vi "Test Write.vi"(8 "error in (no error)":errorcluster, 9 "data table":T1, 10 "data dictionary":refnum<class "data dictionary.lvclass">, 11 "runtime in":refnum<class "SystemLink File runtime.lvclass">) -> (0 "error out":errorcluster, 2 "Pass":bool[](array[boolean]), 3 "runtime out":refnum<class "SystemLink File runtime.lvclass">)   [LabVIEW 2015, in "SystemLink File Module tests.lvlib"]
uses:
  SystemLink File Module tests.lvlib
  module/execution/SystemLink File runtime.lvclass
  <vilib>/NI/Tag Bus/table/data table.ctl
  <vilib>/NI/Tag Bus/dictionary/data dictionary.lvclass
  module/execution/SystemLink File runtime.lvclass/SystemLink File runtime.ctl
  <vilib>/Skyline/Tag/Wrapper/Wrapper_class/NI Skyline Tag.lvclass/NI Skyline Tag.ctl
  <vilib>/NI/Tag Bus/dictionary/data dictionary.lvclass/data dictionary.ctl
  <vilib>/NI/Tag Bus/dictionary/lookup polymorphs/locate double.vi
  <vilib>/NI/Tag Bus/table/data polymorphs/write one/write Double.vi
  <vilib>/NI/Tag Bus/dictionary/lookup polymorphs/locate Single.vi
  <vilib>/NI/Tag Bus/table/data polymorphs/write one/write Single.vi
  <vilib>/NI/Tag Bus/dictionary/lookup polymorphs/locate I32.vi
  <vilib>/NI/Tag Bus/table/data polymorphs/write one/write I32.vi
  <vilib>/NI/Tag Bus/dictionary/lookup polymorphs/locate I16.vi
  <vilib>/NI/Tag Bus/table/data polymorphs/write one/write I16.vi
  <vilib>/NI/Tag Bus/dictionary/lookup polymorphs/locate I8.vi
  <vilib>/NI/Tag Bus/table/data polymorphs/write one/write I8.vi
  <vilib>/NI/Tag Bus/dictionary/lookup polymorphs/locate U64.vi
  <vilib>/NI/Tag Bus/table/data polymorphs/write one/write U64.vi
  <vilib>/NI/Tag Bus/dictionary/lookup polymorphs/locate U32.vi
  <vilib>/NI/Tag Bus/table/data polymorphs/write one/write U32.vi
  <vilib>/NI/Tag Bus/dictionary/lookup polymorphs/locate U16.vi
  <vilib>/NI/Tag Bus/table/data polymorphs/write one/write U16.vi
  <vilib>/NI/Tag Bus/dictionary/lookup polymorphs/locate U8.vi
  <vilib>/NI/Tag Bus/table/data polymorphs/write one/write U8.vi
  <vilib>/NI/Tag Bus/dictionary/lookup polymorphs/locate Boolean.vi
  <vilib>/NI/Tag Bus/table/data polymorphs/write one/write Boolean.vi
  <vilib>/NI/Tag Bus/dictionary/lookup polymorphs/locate String.vi
  <vilib>/NI/Tag Bus/table/data polymorphs/write one/write String.vi
  <vilib>/Skyline/Tag/Wrapper/Wrapper_class/Read Tag Path.vi
  <vilib>/NI/Tag Bus/dictionary/search/find data index.vi
  <vilib>/NI/Tag Bus/dictionary/search/search string list.vi
  <vilib>/NI/Tag Bus/dictionary/tag not found.vi
  <vilib>/Skyline/Tag/Wrapper/Wrapper AMQP_class/Open Tag AMQP.vi
  <vilib>/Skyline/Tag/Wrapper/Wrapper_class/Read Tag (DBL).vi
  <vilib>/Skyline/Tag/Wrapper/Wrapper_class/Close Tag (Single).vi
  <vilib>/Skyline/Tag/Wrapper/Wrapper_class/Read Tag (I32).vi
  <vilib>/Skyline/Tag/Wrapper/Wrapper_class/Read Tag (U64).vi
  <vilib>/Skyline/Tag/Wrapper/Wrapper_class/Read Tag (Boolean).vi
  <vilib>/Skyline/Tag/Wrapper/Wrapper_class/Read Tag (String).vi
  <vilib>/Skyline/Tag/Wrapper/Wrapper_class/Read Tag (Timestamp).vi
  <vilib>/Skyline/Tag/Wrapper/Wrapper_class/NI Skyline Tag.lvclass
  <vilib>/NI/Tag Bus/table/data table.lvlib
  <vilib>/Skyline/Tag/Wrapper/Wrapper AMQP_class/NI Skyline Tag AMQP.lvclass
  module/configuration/SystemLink File configuration.lvclass
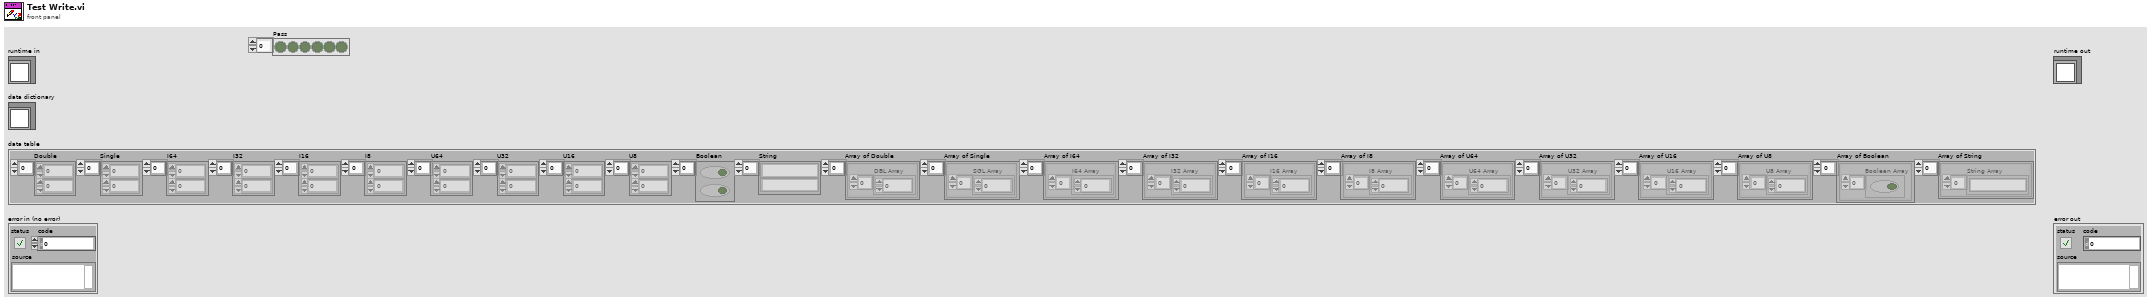
[diagram p1: front panel]
types:
  T1 = typedef "tag bus.lvlib/data table.lvlib/data table.ctl" = cluster{"Double":dbl[], "Single":sgl[], "I64":i64[], "I32":i32[], "I16":i16[], "I8":i8[], "U64":u64[], "U32":u32[], "U16":u16[], "U8":u8[], "Boolean":bool[], "String":string[], "Array of Double":cluster{"DBL Array":dbl[]}[], "Array of Single":cluster{"SGL Array":sgl[]}[], "Array of I64":cluster{"I64 Array":i64[]}[], "Array of I32":cluster{"I32 Array":i32[]}[], "Array of I16":cluster{"I16 Array":i16[]}[], "Array of I8":cluster{"I8 Array":i8[]}[], "Array of U64":cluster{"U64 Array":u64[]}[], "Array of U32":cluster{"U32 Array":u32[]}[], "Array of U16":cluster{"U16 Array":u16[]}[], "Array of U8":cluster{"U8 Array":u8[]}[], "Array of Boolean":cluster{"Boolean Array":bool[]}[], "Array of String":cluster{"String Array":string[]}[]}
  T2 = typedef "SystemLink File configuration.lvclass/SysLink Mapping.ctl" = cluster{"Data Type":T3, "Tag Reference":refnum<class "NI Skyline Tag.lvclass">, "Tag Bus Index":i32, "AMQP":bool, "Skylink Index":i32}
  T3 = typedef "SystemLink File configuration.lvclass/Data Tag Type.ctl" = enum16{"Double", "Single", "I32", "I16", "I8", "U64", "U32", "U16", "U8", "Boolean", "String", "Timestamp"}
  T4 = typedef "NI Skyline Tag.lvlib/DataType.ctl" = enum32{"Double", "I32", "String", "Boolean", "U64", "Timestamp"}
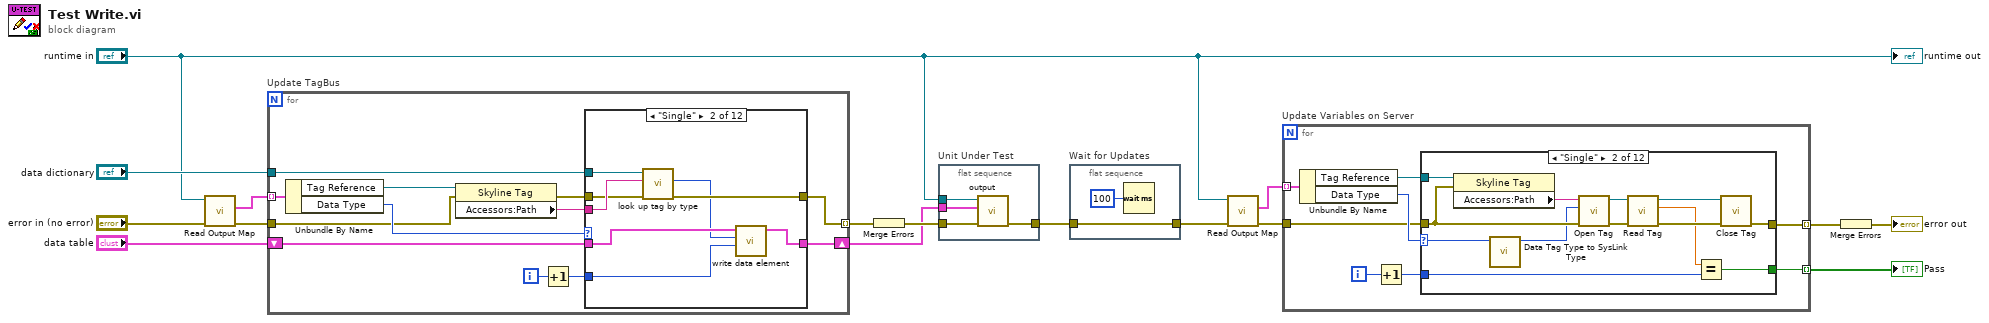
[diagram p0: block diagram]
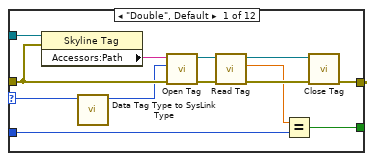
[diagram p2: hidden frame]
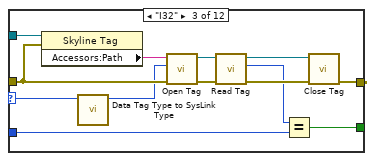
[diagram p3: hidden frame]
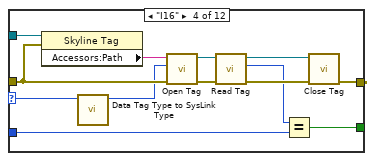
[diagram p4: hidden frame]
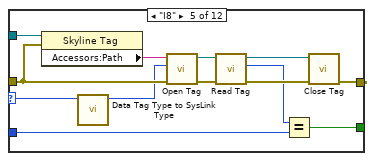
[diagram p5: hidden frame]
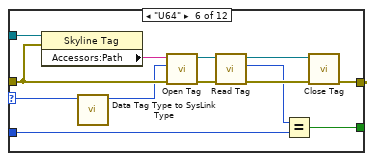
[diagram p6: hidden frame]
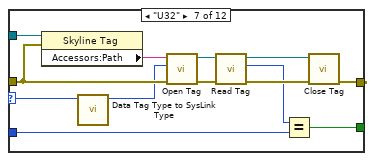
[diagram p7: hidden frame]
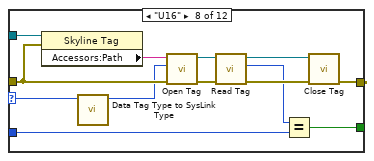
[diagram p8: hidden frame]
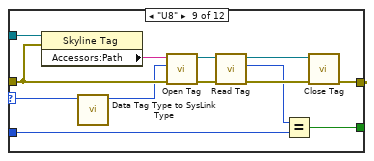
[diagram p9: hidden frame]
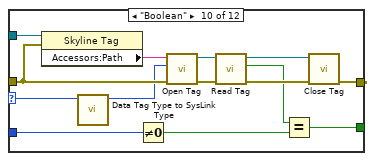
[diagram p10: hidden frame]
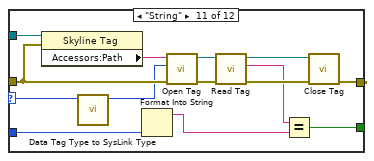
[diagram p11: hidden frame]
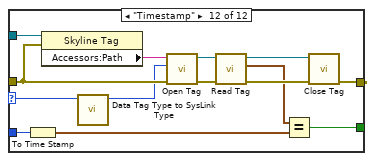
[diagram p12: hidden frame]
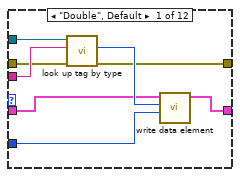
[diagram p13: hidden frame]
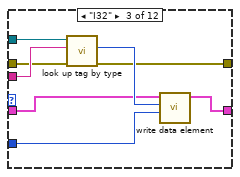
[diagram p14: hidden frame]
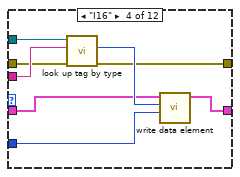
[diagram p15: hidden frame]
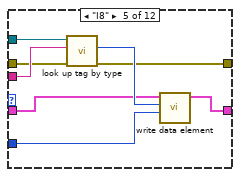
[diagram p16: hidden frame]
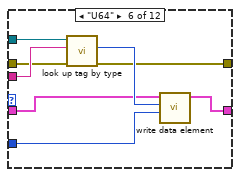
[diagram p17: hidden frame]
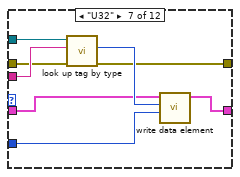
[diagram p18: hidden frame]
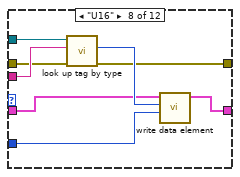
[diagram p19: hidden frame]
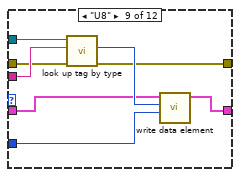
[diagram p20: hidden frame]
diagram:
  n1 = call "Read Output Map.vi"("error in (no error)"="error in (no error)", "SystemLink runtime in"="runtime in") -> ("error out"=w14:errorcluster, "Output"=w15:T2[])  [unwired: 7 in, 1 out]
  n2 = for "Update TagBus" {
    tunnel: w15 -> [w28] mode=indexing
    tunnel: "data dictionary" -> [w25]
    tunnel: w14 -> [w23]
    tunnel: [w18] -> w11 mode=indexing
    shift-right: [w17] -> w9
    shift-left: "data table" -> [w27]
    i -> [w20]
    n3 = Unbundle By Name(w28) -> ("Tag Reference"=w24:refnum<class "NI Skyline Tag.lvclass">, "Data Type"=w26:T3)
    n4 = property class="Skyline Tag"(reference=w24, error in=w23) -> (error out=w22:errorcluster, "Accessors:Path"=w21:string)  [unwired: 1 out]
    n5 = Increment(x=w20) -> (x+1=w19:i32)
    n6 = case shown="\"Single\"" w26 {
      tunnel: w22 -> [w34 w42 w50 w58 w66 w74 w82 w90 w98 w107 w116 w126]
      tunnel: w27 -> [w32 w41 w48 w56 w64 w72 w80 w88 w96 w105 w114 w124]
      tunnel: w25 -> [w36 w44 w52 w60 w68 w76 w84 w92 w100 w109 w118 w128]
      tunnel: w21 -> [w35 w43 w51 w59 w67 w75 w83 w91 w99 w108 w117 w127]
      tunnel: w19 -> [w30 w39 w46 w54 w62 w70 w78 w86 w94 w103 w111 w121]
      tunnel: [w31 w40 w47 w55 w63 w71 w79 w87 w95 w104 w113 w123] -> w18
      tunnel: [w29 w38 w45 w53 w61 w69 w77 w85 w93 w102 w112 w122] -> w17
      frame "Double", Default {
        n7 = call-poly <vilib>:"look up tag by type.vi"("error in"=w34, "name"=w35, "data dictionary in"=w36) -> ("error out"=w31:errorcluster, "index"=w33:i32)  [unwired: 6 in, 1 out]
        n8 = call-poly <vilib>:"write data element.vi"("value"=w30, "index"=w33, "data table in"=w32) -> ("data table out"=w29:T1)  [unwired: 8 in]
      }
      frame "Single" {
        n9 = call-poly <vilib>:"look up tag by type.vi"("error in"=w42, "name"=w43, "data dictionary in"=w44) -> ("error out"=w40:errorcluster, "index"=w37:i32)  [unwired: 6 in, 1 out]
        n10 = call-poly <vilib>:"write data element.vi"("value"=w39, "index"=w37, "data table in"=w41) -> ("data table out"=w38:T1)  [unwired: 8 in]
      }
      frame "I32" {
        n11 = call-poly <vilib>:"look up tag by type.vi"("error in"=w50, "name"=w51, "data dictionary in"=w52) -> ("error out"=w47:errorcluster, "index"=w49:i32)  [unwired: 6 in, 1 out]
        n12 = call-poly <vilib>:"write data element.vi"("value"=w46, "index"=w49, "data table in"=w48) -> ("data table out"=w45:T1)  [unwired: 8 in]
      }
      frame "I16" {
        n13 = call-poly <vilib>:"look up tag by type.vi"("error in"=w58, "name"=w59, "data dictionary in"=w60) -> ("error out"=w55:errorcluster, "index"=w57:i32)  [unwired: 6 in, 1 out]
        n14 = call-poly <vilib>:"write data element.vi"("value"=w54, "index"=w57, "data table in"=w56) -> ("data table out"=w53:T1)  [unwired: 8 in]
      }
      frame "I8" {
        n15 = call-poly <vilib>:"look up tag by type.vi"("error in"=w66, "name"=w67, "data dictionary in"=w68) -> ("error out"=w63:errorcluster, "index"=w65:i32)  [unwired: 6 in, 1 out]
        n16 = call-poly <vilib>:"write data element.vi"("value"=w62, "index"=w65, "data table in"=w64) -> ("data table out"=w61:T1)  [unwired: 8 in]
      }
      frame "U64" {
        n17 = call-poly <vilib>:"look up tag by type.vi"("error in"=w74, "name"=w75, "data dictionary in"=w76) -> ("error out"=w71:errorcluster, "index"=w73:i32)  [unwired: 6 in, 1 out]
        n18 = call-poly <vilib>:"write data element.vi"("value"=w70, "index"=w73, "data table in"=w72) -> ("data table out"=w69:T1)  [unwired: 8 in]
      }
      frame "U32" {
        n19 = call-poly <vilib>:"look up tag by type.vi"("error in"=w82, "name"=w83, "data dictionary in"=w84) -> ("error out"=w79:errorcluster, "index"=w81:i32)  [unwired: 6 in, 1 out]
        n20 = call-poly <vilib>:"write data element.vi"("value"=w78, "index"=w81, "data table in"=w80) -> ("data table out"=w77:T1)  [unwired: 8 in]
      }
      frame "U16" {
        n21 = call-poly <vilib>:"look up tag by type.vi"("error in"=w90, "name"=w91, "data dictionary in"=w92) -> ("error out"=w87:errorcluster, "index"=w89:i32)  [unwired: 6 in, 1 out]
        n22 = call-poly <vilib>:"write data element.vi"("value"=w86, "index"=w89, "data table in"=w88) -> ("data table out"=w85:T1)  [unwired: 8 in]
      }
      frame "U8" {
        n23 = call-poly <vilib>:"look up tag by type.vi"("error in"=w98, "name"=w99, "data dictionary in"=w100) -> ("error out"=w95:errorcluster, "index"=w97:i32)  [unwired: 6 in, 1 out]
        n24 = call-poly <vilib>:"write data element.vi"("value"=w94, "index"=w97, "data table in"=w96) -> ("data table out"=w93:T1)  [unwired: 8 in]
      }
      frame "Boolean" {
        n25 = Not Equal To 0?(x=w103) -> (x != 0?=w101:bool)
        n26 = call-poly <vilib>:"look up tag by type.vi"("error in"=w107, "name"=w108, "data dictionary in"=w109) -> ("error out"=w104:errorcluster, "index"=w106:i32)  [unwired: 6 in, 1 out]
        n27 = call-poly <vilib>:"write data element.vi"("value"=w101, "index"=w106, "data table in"=w105) -> ("data table out"=w102:T1)  [unwired: 8 in]
      }
      frame "String" {
        n28 = call-poly <vilib>:"look up tag by type.vi"("error in"=w116, "name"=w117, "data dictionary in"=w118) -> ("error out"=w113:errorcluster, "index"=w115:i32)  [unwired: 6 in, 1 out]
        n29 = Format Into String(w111) -> (resulting string=w110:string)  [unwired: 3 in, 1 out]
        n30 = call-poly <vilib>:"write data element.vi"("value"=w110, "index"=w115, "data table in"=w114) -> ("data table out"=w112:T1)  [unwired: 8 in]
      }
      frame "Timestamp" {
        n31 = To Time Stamp(1:w121) -> (0:w120:timestamp)
        n32 = call-poly <vilib>:"look up tag by type.vi"("error in"=w126, "name"=w127, "data dictionary in"=w128) -> ("error out"=w123:errorcluster, "index"=w125:i32)  [unwired: 6 in, 1 out]
        n33 = To Double Precision Float(number=w120) -> (double precision float=w119:dbl)
        n34 = call-poly <vilib>:"write data element.vi"("value"=w119, "index"=w125, "data table in"=w124) -> ("data table out"=w122:T1)  [unwired: 8 in]
      }
    }
  }
  n35 = Merge Errors(w11) -> (w10:errorcluster)
  n36 = flat-sequence "Unit Under Test" {
    tunnel: w10 -> [w132]
    tunnel: w9 -> [w131]
    tunnel: "runtime in" -> [w130]
    tunnel: [w129] -> w8
    frame #0 {
      n37 = call-dynamic "output.vi"("error in"=w132, "data table in"=w131, "SystemLin Tag Module runtime in"=w130) -> ("error out"=w129:errorcluster)  [unwired: 6 in, 2 out]
    }
  }
  n38 = flat-sequence "Wait for Updates" {
    tunnel: [w133] -> w7
    tunnel: w8 -> [w133]
    frame #0 {
      n39 = Wait (ms)(milliseconds to wait=u32 100) -> ()  [unwired: 1 out]
    }
  }
  n40 = call "Read Output Map.vi"("error in (no error)"=w7, "SystemLink runtime in"="runtime in") -> ("error out"=w6:errorcluster, "Output"=w5:T2[])  [unwired: 7 in, 1 out]
  n41 = for "Update Variables on Server" {
    tunnel: w5 -> [w142] mode=indexing
    tunnel: w6 -> [w139]
    tunnel: [w136] -> w3 mode=indexing
    tunnel: [w135] -> w1 mode=indexing
    i -> [w138]
    n42 = Unbundle By Name(w142) -> ("Tag Reference"=w140:refnum<class "NI Skyline Tag.lvclass">, "Data Type"=w141:T3)
    n43 = Increment(x=w138) -> (x+1=w137:i32)
    n44 = case shown="\"Single\"" w141 {
      selector: w141 -> [w152 w165 w178 w191 w204 w217 w230 w243 w256 w270 w284 w298]
      tunnel: w140 -> [w155 w168 w181 w194 w207 w220 w233 w246 w259 w273 w287 w301]
      tunnel: w139 -> [w153 w166 w179 w192 w205 w218 w231 w244 w257 w271 w285 w299]
      tunnel: w137 -> [w145 w158 w171 w184 w197 w210 w223 w236 w249 w263 w275 w289]
      tunnel: [w146 w159 w172 w185 w198 w211 w224 w237 w250 w264 w278 w292] -> w136
      tunnel: [w143 w156 w169 w182 w195 w208 w221 w234 w247 w261 w276 w290] -> w135
      frame "Double", Default {
        n45 = property class="Skyline Tag"(reference=w155, error in=w153) -> ("Accessors:Path"=w154:string)  [unwired: 2 out]
        n46 = call "Data Tag Type to SysLink Type.vi"("Data Tag Type"=w152) -> ("data type"=w151:T4)  [unwired: 10 in]
        n47 = call-poly <vilib>:"Open Tag.vi"("error in (no error)"=w153, "data type"=w151, "path"=w154) -> ("error out"=w149:errorcluster, "tag out"=w150:refnum<class "NI Skyline Tag.lvclass">)  [unwired: 7 in]
        n48 = call-poly <vilib>:"Read Tag.vi"("error in (no error)"=w149, "tag in"=w150) -> ("error out"=w147:errorcluster, "value"=w144:dbl, "tag out"=w148:refnum<class "NI Skyline Tag.lvclass">)  [unwired: 5 in, 2 out]
        n49 = Equal?(x=w144, y=w145) -> (x = y?=w143:bool)
        n50 = call-poly <vilib>:"Close Tag.vi"("error in (no error)"=w147, "tag in"=w148) -> ("error out"=w146:errorcluster)  [unwired: 9 in]
      }
      frame "Single" {
        n51 = property class="Skyline Tag"(reference=w168, error in=w166) -> ("Accessors:Path"=w167:string)  [unwired: 2 out]
        n52 = call "Data Tag Type to SysLink Type.vi"("Data Tag Type"=w165) -> ("data type"=w164:T4)  [unwired: 10 in]
        n53 = call-poly <vilib>:"Open Tag.vi"("error in (no error)"=w166, "data type"=w164, "path"=w167) -> ("error out"=w162:errorcluster, "tag out"=w163:refnum<class "NI Skyline Tag.lvclass">)  [unwired: 7 in]
        n54 = call-poly <vilib>:"Read Tag.vi"("error in (no error)"=w162, "tag in"=w163) -> ("error out"=w160:errorcluster, "value"=w157:dbl, "tag out"=w161:refnum<class "NI Skyline Tag.lvclass">)  [unwired: 5 in, 2 out]
        n55 = Equal?(x=w157, y=w158) -> (x = y?=w156:bool)
        n56 = call-poly <vilib>:"Close Tag.vi"("error in (no error)"=w160, "tag in"=w161) -> ("error out"=w159:errorcluster)  [unwired: 9 in]
      }
      frame "I32" {
        n57 = property class="Skyline Tag"(reference=w181, error in=w179) -> ("Accessors:Path"=w180:string)  [unwired: 2 out]
        n58 = call "Data Tag Type to SysLink Type.vi"("Data Tag Type"=w178) -> ("data type"=w177:T4)  [unwired: 10 in]
        n59 = call-poly <vilib>:"Open Tag.vi"("error in (no error)"=w179, "data type"=w177, "path"=w180) -> ("error out"=w175:errorcluster, "tag out"=w176:refnum<class "NI Skyline Tag.lvclass">)  [unwired: 7 in]
        n60 = call-poly <vilib>:"Read Tag.vi"("error in (no error)"=w175, "tag in"=w176) -> ("error out"=w173:errorcluster, "value"=w170:i32, "tag out"=w174:refnum<class "NI Skyline Tag.lvclass">)  [unwired: 5 in, 2 out]
        n61 = Equal?(x=w170, y=w171) -> (x = y?=w169:bool)
        n62 = call-poly <vilib>:"Close Tag.vi"("error in (no error)"=w173, "tag in"=w174) -> ("error out"=w172:errorcluster)  [unwired: 9 in]
      }
      frame "I16" {
        n63 = property class="Skyline Tag"(reference=w194, error in=w192) -> ("Accessors:Path"=w193:string)  [unwired: 2 out]
        n64 = call "Data Tag Type to SysLink Type.vi"("Data Tag Type"=w191) -> ("data type"=w190:T4)  [unwired: 10 in]
        n65 = call-poly <vilib>:"Open Tag.vi"("error in (no error)"=w192, "data type"=w190, "path"=w193) -> ("error out"=w188:errorcluster, "tag out"=w189:refnum<class "NI Skyline Tag.lvclass">)  [unwired: 7 in]
        n66 = call-poly <vilib>:"Read Tag.vi"("error in (no error)"=w188, "tag in"=w189) -> ("error out"=w186:errorcluster, "value"=w183:i32, "tag out"=w187:refnum<class "NI Skyline Tag.lvclass">)  [unwired: 5 in, 2 out]
        n67 = Equal?(x=w183, y=w184) -> (x = y?=w182:bool)
        n68 = call-poly <vilib>:"Close Tag.vi"("error in (no error)"=w186, "tag in"=w187) -> ("error out"=w185:errorcluster)  [unwired: 9 in]
      }
      frame "I8" {
        n69 = property class="Skyline Tag"(reference=w207, error in=w205) -> ("Accessors:Path"=w206:string)  [unwired: 2 out]
        n70 = call "Data Tag Type to SysLink Type.vi"("Data Tag Type"=w204) -> ("data type"=w203:T4)  [unwired: 10 in]
        n71 = call-poly <vilib>:"Open Tag.vi"("error in (no error)"=w205, "data type"=w203, "path"=w206) -> ("error out"=w201:errorcluster, "tag out"=w202:refnum<class "NI Skyline Tag.lvclass">)  [unwired: 7 in]
        n72 = call-poly <vilib>:"Read Tag.vi"("error in (no error)"=w201, "tag in"=w202) -> ("error out"=w199:errorcluster, "value"=w196:i32, "tag out"=w200:refnum<class "NI Skyline Tag.lvclass">)  [unwired: 5 in, 2 out]
        n73 = Equal?(x=w196, y=w197) -> (x = y?=w195:bool)
        n74 = call-poly <vilib>:"Close Tag.vi"("error in (no error)"=w199, "tag in"=w200) -> ("error out"=w198:errorcluster)  [unwired: 9 in]
      }
      frame "U64" {
        n75 = property class="Skyline Tag"(reference=w220, error in=w218) -> ("Accessors:Path"=w219:string)  [unwired: 2 out]
        n76 = call "Data Tag Type to SysLink Type.vi"("Data Tag Type"=w217) -> ("data type"=w216:T4)  [unwired: 10 in]
        n77 = call-poly <vilib>:"Open Tag.vi"("error in (no error)"=w218, "data type"=w216, "path"=w219) -> ("error out"=w214:errorcluster, "tag out"=w215:refnum<class "NI Skyline Tag.lvclass">)  [unwired: 7 in]
        n78 = call-poly <vilib>:"Read Tag.vi"("error in (no error)"=w214, "tag in"=w215) -> ("error out"=w212:errorcluster, "value"=w209:u64, "tag out"=w213:refnum<class "NI Skyline Tag.lvclass">)  [unwired: 5 in, 2 out]
        n79 = Equal?(x=w209, y=w210) -> (x = y?=w208:bool)
        n80 = call-poly <vilib>:"Close Tag.vi"("error in (no error)"=w212, "tag in"=w213) -> ("error out"=w211:errorcluster)  [unwired: 9 in]
      }
      frame "U32" {
        n81 = property class="Skyline Tag"(reference=w233, error in=w231) -> ("Accessors:Path"=w232:string)  [unwired: 2 out]
        n82 = call "Data Tag Type to SysLink Type.vi"("Data Tag Type"=w230) -> ("data type"=w229:T4)  [unwired: 10 in]
        n83 = call-poly <vilib>:"Open Tag.vi"("error in (no error)"=w231, "data type"=w229, "path"=w232) -> ("error out"=w227:errorcluster, "tag out"=w228:refnum<class "NI Skyline Tag.lvclass">)  [unwired: 7 in]
        n84 = call-poly <vilib>:"Read Tag.vi"("error in (no error)"=w227, "tag in"=w228) -> ("error out"=w225:errorcluster, "value"=w222:u64, "tag out"=w226:refnum<class "NI Skyline Tag.lvclass">)  [unwired: 5 in, 2 out]
        n85 = Equal?(x=w222, y=w223) -> (x = y?=w221:bool)
        n86 = call-poly <vilib>:"Close Tag.vi"("error in (no error)"=w225, "tag in"=w226) -> ("error out"=w224:errorcluster)  [unwired: 9 in]
      }
      frame "U16" {
        n87 = property class="Skyline Tag"(reference=w246, error in=w244) -> ("Accessors:Path"=w245:string)  [unwired: 2 out]
        n88 = call "Data Tag Type to SysLink Type.vi"("Data Tag Type"=w243) -> ("data type"=w242:T4)  [unwired: 10 in]
        n89 = call-poly <vilib>:"Open Tag.vi"("error in (no error)"=w244, "data type"=w242, "path"=w245) -> ("error out"=w240:errorcluster, "tag out"=w241:refnum<class "NI Skyline Tag.lvclass">)  [unwired: 7 in]
        n90 = call-poly <vilib>:"Read Tag.vi"("error in (no error)"=w240, "tag in"=w241) -> ("error out"=w238:errorcluster, "value"=w235:u64, "tag out"=w239:refnum<class "NI Skyline Tag.lvclass">)  [unwired: 5 in, 2 out]
        n91 = Equal?(x=w235, y=w236) -> (x = y?=w234:bool)
        n92 = call-poly <vilib>:"Close Tag.vi"("error in (no error)"=w238, "tag in"=w239) -> ("error out"=w237:errorcluster)  [unwired: 9 in]
      }
      frame "U8" {
        n93 = property class="Skyline Tag"(reference=w259, error in=w257) -> ("Accessors:Path"=w258:string)  [unwired: 2 out]
        n94 = call "Data Tag Type to SysLink Type.vi"("Data Tag Type"=w256) -> ("data type"=w255:T4)  [unwired: 10 in]
        n95 = call-poly <vilib>:"Open Tag.vi"("error in (no error)"=w257, "data type"=w255, "path"=w258) -> ("error out"=w253:errorcluster, "tag out"=w254:refnum<class "NI Skyline Tag.lvclass">)  [unwired: 7 in]
        n96 = call-poly <vilib>:"Read Tag.vi"("error in (no error)"=w253, "tag in"=w254) -> ("error out"=w251:errorcluster, "value"=w248:u64, "tag out"=w252:refnum<class "NI Skyline Tag.lvclass">)  [unwired: 5 in, 2 out]
        n97 = Equal?(x=w248, y=w249) -> (x = y?=w247:bool)
        n98 = call-poly <vilib>:"Close Tag.vi"("error in (no error)"=w251, "tag in"=w252) -> ("error out"=w250:errorcluster)  [unwired: 9 in]
      }
      frame "Boolean" {
        n99 = property class="Skyline Tag"(reference=w273, error in=w271) -> ("Accessors:Path"=w272:string)  [unwired: 2 out]
        n100 = call "Data Tag Type to SysLink Type.vi"("Data Tag Type"=w270) -> ("data type"=w269:T4)  [unwired: 10 in]
        n101 = Not Equal To 0?(x=w263) -> (x != 0?=w260:bool)
        n102 = call-poly <vilib>:"Open Tag.vi"("error in (no error)"=w271, "data type"=w269, "path"=w272) -> ("error out"=w267:errorcluster, "tag out"=w268:refnum<class "NI Skyline Tag.lvclass">)  [unwired: 7 in]
        n103 = call-poly <vilib>:"Read Tag.vi"("error in (no error)"=w267, "tag in"=w268) -> ("error out"=w265:errorcluster, "value"=w262:bool, "tag out"=w266:refnum<class "NI Skyline Tag.lvclass">)  [unwired: 5 in, 2 out]
        n104 = Equal?(x=w262, y=w260) -> (x = y?=w261:bool)
        n105 = call-poly <vilib>:"Close Tag.vi"("error in (no error)"=w265, "tag in"=w266) -> ("error out"=w264:errorcluster)  [unwired: 9 in]
      }
      frame "String" {
        n106 = property class="Skyline Tag"(reference=w287, error in=w285) -> ("Accessors:Path"=w286:string)  [unwired: 2 out]
        n107 = call "Data Tag Type to SysLink Type.vi"("Data Tag Type"=w284) -> ("data type"=w283:T4)  [unwired: 10 in]
        n108 = Format Into String(w275) -> (resulting string=w274:string)  [unwired: 3 in, 1 out]
        n109 = call-poly <vilib>:"Open Tag.vi"("error in (no error)"=w285, "data type"=w283, "path"=w286) -> ("error out"=w281:errorcluster, "tag out"=w282:refnum<class "NI Skyline Tag.lvclass">)  [unwired: 7 in]
        n110 = call-poly <vilib>:"Read Tag.vi"("error in (no error)"=w281, "tag in"=w282) -> ("error out"=w279:errorcluster, "value"=w277:string, "tag out"=w280:refnum<class "NI Skyline Tag.lvclass">)  [unwired: 5 in, 2 out]
        n111 = Equal?(x=w277, y=w274) -> (x = y?=w276:bool)
        n112 = call-poly <vilib>:"Close Tag.vi"("error in (no error)"=w279, "tag in"=w280) -> ("error out"=w278:errorcluster)  [unwired: 9 in]
      }
      frame "Timestamp" {
        n113 = To Time Stamp(1:w289) -> (0:w288:timestamp)
        n114 = property class="Skyline Tag"(reference=w301, error in=w299) -> ("Accessors:Path"=w300:string)  [unwired: 2 out]
        n115 = call "Data Tag Type to SysLink Type.vi"("Data Tag Type"=w298) -> ("data type"=w297:T4)  [unwired: 10 in]
        n116 = call-poly <vilib>:"Open Tag.vi"("error in (no error)"=w299, "data type"=w297, "path"=w300) -> ("error out"=w295:errorcluster, "tag out"=w296:refnum<class "NI Skyline Tag.lvclass">)  [unwired: 7 in]
        n117 = call-poly <vilib>:"Read Tag.vi"("error in (no error)"=w295, "tag in"=w296) -> ("error out"=w293:errorcluster, "value"=w291:timestamp, "tag out"=w294:refnum<class "NI Skyline Tag.lvclass">)  [unwired: 5 in, 2 out]
        n118 = Equal?(x=w291, y=w288) -> (x = y?=w290:bool)
        n119 = call-poly <vilib>:"Close Tag.vi"("error in (no error)"=w293, "tag in"=w294) -> ("error out"=w292:errorcluster)  [unwired: 9 in]
      }
    }
  }
  "Pass" <- w1
  n120 = Merge Errors(w3) -> (→"error out":errorcluster)
  "runtime out" <- "runtime in"
